vi "rndTempGen.vi"() -> (3 "Numeric":i32)   [LabVIEW 2017]
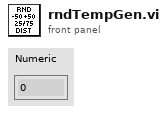
[diagram p1: front panel]
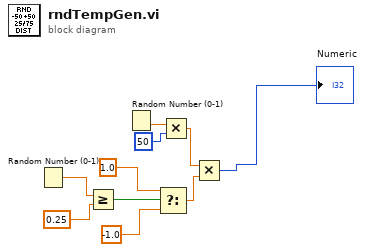
[diagram p0: block diagram]
diagram:
  n1 = Random Number (0-1)() -> (number: 0 to 1=w1:dbl)
  n2 = Greater Or Equal?(x=w1, y=0.25) -> (x >= y?=w5:bool)
  n3 = Random Number (0-1)() -> (number: 0 to 1=w6:dbl)
  n4 = Select(t=1.0, s=w5, f=-1.0) -> (s? t:f=w8:dbl)
  n5 = Multiply(x=w6, y=50) -> (x*y=w7:dbl)
  n6 = Multiply(x=w7, y=w8) -> (x*y=→"Numeric":i32)
